vi "SVFA FFT Spectrum (Mag-Phase).vi"   [LabVIEW 2017]
doc: "Computes the Fast Fourier Transform (FFT) spectrum of <B>scaled signal [EU]</B>. This VI returns FFT results as the magnitude and phase of the FFT spectrum. Wire data to the <B>scaled signal [EU]</B> input to determine the polymorphic instance to use or manually select the instance."
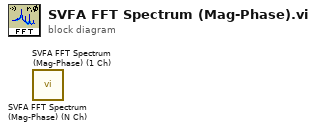
[diagram p0: block diagram]
diagram:
  n1 = call <vilib>:"SVFA FFT Spectrum (Mag-Phase) (N Ch).vi"() -> ()  [unwired: 12 in, 8 out]
  n2 = call <vilib>:"SVFA FFT Spectrum (Mag-Phase) (1 Ch).vi"() -> ()  [unwired: 12 in, 8 out]
